vi "Read Gates From Registry (Internal).vi"(8 "error in (no error)":errorcluster, 9 "dt (us)":dbl, 10 "CMD LUT":variant, 11 "Test No.":u32) -> (0 "error out":errorcluster, 2 "Gates":T1={"Display Gate"={"Start"=0.0, "Length"=100.0}, "ETM Mode"=enum."Echo Trigger OFF", "Echo Gate"={"Start (us)"=0.0, "Length (us)"=100.0, "Threshold"=10, "Colour"=0}, "Insp Gates"=[]} {"Insp Gates"."Max # Peaks" max=64000 step=100; "Insp Gates"."Threshold" min=10 max=4095 step=10; "Insp Gates"."Length (us)" min=0.0 max=96000.0 step=100.0; "Insp Gates"."Start (us)" min=0.0 max=64000.0 step=100.0; "Echo Gate"."Threshold" min=10 max=4095 step=10; "Echo Gate"."Length (us)" min=0.0 max=96000.0 step=100.0; "Echo Gate"."Start (us)" min=0.0 max=64000.0 step=100.0; "Display Gate"."Length" min=0.0 max=64000.0 step=1000.0; "Display Gate"."Start" min=0.0 max=64000.0 step=1000.0})   [LabVIEW 2026, in "MicroPulse_Driver.lvlib"]
uses:
  MicroPulse_Driver.lvlib
  Public/Data/Datatypes/subdatatypes/MP - Registry Gates.ctl
  Public/Data/Datatypes/MP - display gate.ctl
  Public/Data/Datatypes/MP - echo gate mode.ctl
  Public/Data/Datatypes/MP - echo gate parameters.ctl
  Public/Data/Datatypes/MP - multigate inspection gate parameters.ctl
  Public/Data/Datatypes/MP - hysteresis level.ctl
  Public/Data/Datatypes/MP - multigate mode.ctl
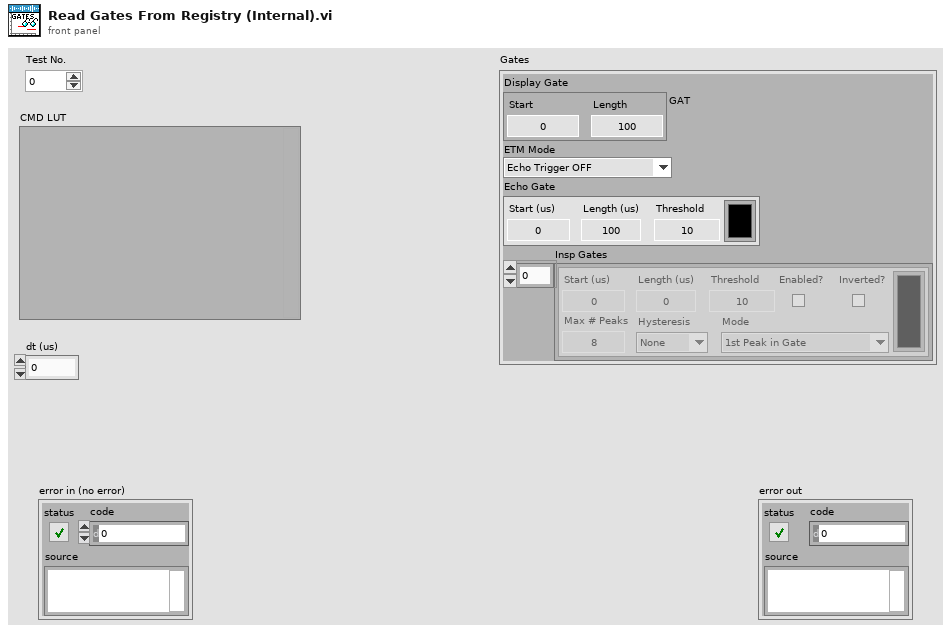
[diagram p1: front panel]
types:
  T1 = typedef "MicroPulse_Driver.lvlib/MP - Registry Gates.ctl" = cluster{"Display Gate":T2, "ETM Mode":T3, "Echo Gate":T4, "Insp Gates":T5[]}
  T2 = typedef "MicroPulse_Driver.lvlib/MP - display gate.ctl" = cluster{"Start":dbl, "Length":dbl}
  T3 = typedef "MicroPulse_Driver.lvlib/MP - echo gate mode.ctl" = enum16{"Echo Trigger OFF", "Echo Gate Display Mode", "Echo Trigger ON", "Multi Gate or FMC Mode", "Reserved", "PA - Echo Trigger ON"}
  T4 = typedef "MicroPulse_Driver.lvlib/MP - echo gate parameters.ctl" = cluster{"Start (us)":dbl, "Length (us)":dbl, "Threshold":u16, "Colour":u32}
  T5 = typedef "MicroPulse_Driver.lvlib/MP - multigate inspection gate parameters.ctl" = cluster{"Start (us)":dbl, "Length (us)":dbl, "Threshold":u16, "Enabled?":bool, "Max # Peaks":u16, "Hysteresis":T6, "Mode":T7, "Inverted?":bool, "Colour ":u32}
  T6 = typedef "MicroPulse_Driver.lvlib/MP - hysteresis level.ctl" = enum16{"None", "3dB", "6dB", "9dB", "12dB"}
  T7 = typedef "MicroPulse_Driver.lvlib/MP - multigate mode.ctl" = enum16{"1st Peak in Gate", "Largest Peak In Gate", "All Peaks In Gate", "1st Threshold Crossing"}
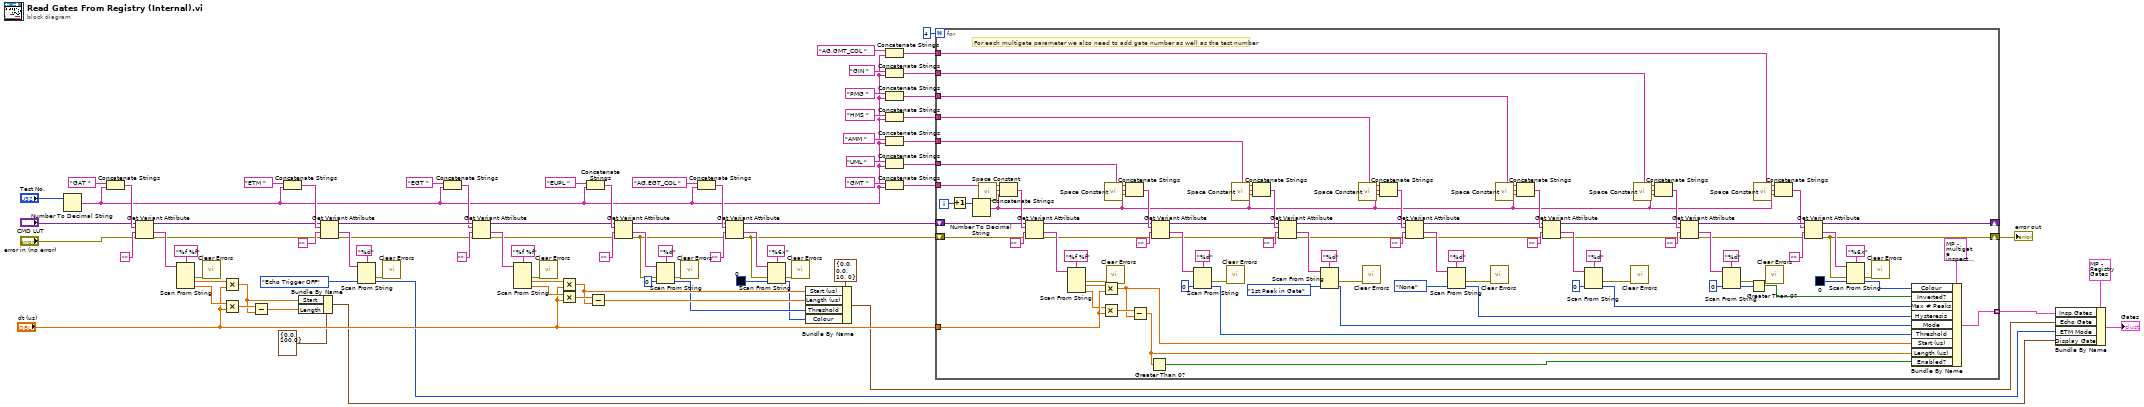
[diagram p0: block diagram]
diagram:
  n1 = Number To Decimal String(number="Test No.") -> (decimal integer string=w6:string)  [unwired: 1 in]
  n2 = Concatenate Strings("GAT " ("name"), w6) -> (w32:string)
  n3 = Get Variant Attribute(Variant="CMD LUT", name=w32, default value (empty Variant)="", error in="error in (no error)") -> (duplicate Variant=w16:variant, value=w34:string, error out=w18:errorcluster)  [unwired: 1 out]
  n4 = Scan From String(format string="%f %f", input string=w34) -> (error out=w38:errorcluster, output 1=w35:dbl, output 2=w36:dbl)  [unwired: 4 in, 2 out]
  n5 = call <vilib>:"Clear Errors.vi"("error in (no error)"=w38) -> ()  [unwired: 5 in, 2 out]
  n6 = Multiply(x=w35, y="dt (us)") -> (x*y=w27:dbl)
  n7 = Multiply(x=w36, y="dt (us)") -> (x*y=w37:dbl)
  n8 = Subtract(x=w37, y=w27) -> (x-y=w26:dbl)
  n9 = Concatenate Strings("ETM " ("name"), w6) -> (w76:string)
  n10 = Bundle By Name(cluster=T2 {"Start"=0.0, "Length"=100.0} ("Display Gate"), "Start"=w27, "Length"=w26) -> (w20:T2)
  n11 = Get Variant Attribute(Variant=w16, name=w76, default value (empty Variant)="", error in=w18) -> (duplicate Variant=w79:variant, value=w82:string, error out=w41:errorcluster)  [unwired: 1 out]
  n12 = Scan From String(format string="%d", input string=w82, default 1=MP_-_echo_gate_mode."Echo Trigger OFF" ("Echo Gate Mode")) -> (error out=w40:errorcluster, output 1=w21:T3)  [unwired: 2 in, 2 out]
  n13 = call <vilib>:"Clear Errors.vi"("error in (no error)"=w40) -> ()  [unwired: 5 in, 2 out]
  n14 = Concatenate Strings("EGT " ("name"), w6) -> (w74:string)
  n15 = Get Variant Attribute(Variant=w79, name=w74, default value (empty Variant)="", error in=w41) -> (duplicate Variant=w58:variant, value=w72:string, error out=w42:errorcluster)  [unwired: 1 out]
  n16 = Scan From String(format string="%f %f", input string=w72) -> (error out=w39:errorcluster, output 1=w65:dbl, output 2=w64:dbl)  [unwired: 4 in, 2 out]
  n17 = call <vilib>:"Clear Errors.vi"("error in (no error)"=w39) -> ()  [unwired: 5 in, 2 out]
  n18 = Multiply(x=w65, y="dt (us)") -> (x*y=w60:dbl)
  n19 = Multiply(x=w64, y="dt (us)") -> (x*y=w63:dbl)
  n20 = Concatenate Strings("EUPL " ("name"), w6) -> (w69:string)
  n21 = Subtract(x=w63, y=w60) -> (x-y=w61:dbl)
  n22 = Get Variant Attribute(Variant=w58, name=w69, default value (empty Variant)="", error in=w42) -> (duplicate Variant=w4:variant, value=w71:string, error out=w2:errorcluster)  [unwired: 1 out]
  n23 = Scan From String(format string="%d", input string=w71, error in=w2, default 1=u16 0 ("default value 1")) -> (error out=w54:errorcluster, output 1=w59:u16)  [unwired: 1 in, 2 out]
  n24 = call <vilib>:"Clear Errors.vi"("error in (no error)"=w54) -> ()  [unwired: 5 in, 2 out]
  n25 = Concatenate Strings("AG.EGT_COL " ("name"), w6) -> (w12:string)
  n26 = Get Variant Attribute(Variant=w4, name=w12, default value (empty Variant)="", error in=w2) -> (duplicate Variant=w3:variant, value=w10:string, error out=w1:errorcluster)  [unwired: 1 out]
  n27 = Scan From String(format string="%6x", input string=w10, error in=w1, default 1=u32 0 ("Color Box")) -> (error out=w15:errorcluster, output 1=w9:u32)  [unwired: 1 in, 2 out]
  n28 = call <vilib>:"Clear Errors.vi"("error in (no error)"=w15) -> ()  [unwired: 5 in, 2 out]
  n29 = Bundle By Name(cluster=T4 {"Start (us)"=0.0, "Length (us)"=0.0, "Threshold"=10, "Colour"=0} ("Echo Gate Parameters"), "Start (us)"=w60, "Length (us)"=w61, "Threshold"=w59, "Colour"=w9) -> (w22:T4)
  n30 = Concatenate Strings("AG.GMT_COL " ("name"), w6) -> (w5:string)
  n31 = Concatenate Strings("GIN " ("name"), w6) -> (w44:string)
  n32 = Concatenate Strings("PMG " ("name"), w6) -> (w45:string)
  n33 = Concatenate Strings("HMS " ("name"), w6) -> (w46:string)
  n34 = Concatenate Strings("AMM " ("name"), w6) -> (w50:string)
  n35 = Concatenate Strings("UML " ("name"), w6) -> (w52:string)
  n36 = Concatenate Strings("GMT " ("name"), w6) -> (w56:string)
  n37 = for {
    N: 4 -> [_]
    tunnel: w56 -> [w173]
    shift-right: [w92] -> _
    shift-left: w3 -> [w166]
    shift-right: [w90] -> w43
    shift-left: w1 -> [w165]
    tunnel: "dt (us)" -> [w162]
    tunnel: w52 -> [w155]
    tunnel: w50 -> [w147]
    tunnel: w46 -> [w123]
    tunnel: w45 -> [w122]
    tunnel: w44 -> [w121]
    tunnel: [w110] -> w23 mode=indexing
    tunnel: w5 -> [w85]
    i -> [w169]
    # "For each multigate parameter we also need to add gate number as well as the test number"
    n38 = Increment(x=w169) -> (x+1=w168:i32)
    n39 = Number To Decimal String(number=w168) -> (decimal integer string=w86:string)  [unwired: 1 in]
    n40 = call <vilib>:"Space Constant.vi"() -> ("String"=w167:string)
    n41 = Concatenate Strings(w173, w167, w86) -> (w170:string)
    n42 = Get Variant Attribute(Variant=w166, name=w170, default value (empty Variant)="", error in=w165) -> (duplicate Variant=w154:variant, value=w171:string, error out=w109:errorcluster)  [unwired: 1 out]
    n43 = Scan From String(format string="%f %f", input string=w171) -> (error out=w108:errorcluster, output 1=w163:dbl, output 2=w161:dbl)  [unwired: 4 in, 2 out]
    n44 = Multiply(x=w163, y=w162) -> (x*y=w111:dbl)
    n45 = Multiply(x=w161, y=w162) -> (x*y=w164:dbl)
    n46 = call <vilib>:"Space Constant.vi"() -> ("String"=w160:string)
    n47 = call <vilib>:"Clear Errors.vi"("error in (no error)"=w108) -> ()  [unwired: 5 in, 2 out]
    n48 = Concatenate Strings(w155, w160, w86) -> (w156:string)
    n49 = Subtract(x=w164, y=w111) -> (x-y=w112:dbl)
    n50 = Greater Than 0?(x=w112) -> (x > 0?=w113:bool)
    n51 = Get Variant Attribute(Variant=w154, name=w156, default value (empty Variant)="", error in=w109) -> (duplicate Variant=w145:variant, value=w159:string, error out=w100:errorcluster)  [unwired: 1 out]
    n52 = Scan From String(format string="%d", input string=w159, default 1=u16 0 ("default value 1")) -> (error out=w99:errorcluster, output 1=w114:u16)  [unwired: 2 in, 2 out]
    n53 = call <vilib>:"Clear Errors.vi"("error in (no error)"=w99) -> ()  [unwired: 5 in, 2 out]
    n54 = call <vilib>:"Space Constant.vi"() -> ("String"=w148:string)
    n55 = Concatenate Strings(w147, w148, w86) -> (w152:string)
    n56 = Get Variant Attribute(Variant=w145, name=w152, default value (empty Variant)="", error in=w100) -> (duplicate Variant=w127:variant, value=w149:string, error out=w102:errorcluster)  [unwired: 1 out]
    n57 = Scan From String(format string="%d", input string=w149, default 1=MP_-_multigate_mode."1st Peak in Gate" ("Value")) -> (error out=w101:errorcluster, output 1=w115:T7)  [unwired: 2 in, 2 out]
    n58 = call <vilib>:"Space Constant.vi"() -> ("String"=w140:string)
    n59 = call <vilib>:"Clear Errors.vi"("error in (no error)"=w101) -> ()  [unwired: 5 in, 2 out]
    n60 = Concatenate Strings(w123, w140, w86) -> (w144:string)
    n61 = Get Variant Attribute(Variant=w127, name=w144, default value (empty Variant)="", error in=w102) -> (duplicate Variant=w126:variant, value=w141:string, error out=w104:errorcluster)  [unwired: 1 out]
    n62 = Scan From String(format string="%d", input string=w141, default 1=MP_-_hysteresis_level."None" ("Value")) -> (error out=w103:errorcluster, output 1=w116:T6)  [unwired: 2 in, 2 out]
    n63 = call <vilib>:"Clear Errors.vi"("error in (no error)"=w103) -> ()  [unwired: 5 in, 2 out]
    n64 = call <vilib>:"Space Constant.vi"() -> ("String"=w139:string)
    n65 = Concatenate Strings(w122, w139, w86) -> (w135:string)
    n66 = Get Variant Attribute(Variant=w126, name=w135, default value (empty Variant)="", error in=w104) -> (duplicate Variant=w125:variant, value=w138:string, error out=w106:errorcluster)  [unwired: 1 out]
    n67 = Scan From String(format string="%d", input string=w138, default 1=u16 0 ("default value 1")) -> (error out=w105:errorcluster, output 1=w117:u16)  [unwired: 2 in, 2 out]
    n68 = call <vilib>:"Clear Errors.vi"("error in (no error)"=w105) -> ()  [unwired: 5 in, 2 out]
    n69 = call <vilib>:"Space Constant.vi"() -> ("String"=w128:string)
    n70 = Concatenate Strings(w121, w128, w86) -> (w132:string)
    n71 = Get Variant Attribute(Variant=w125, name=w132, default value (empty Variant)="", error in=w106) -> (duplicate Variant=w93:variant, value=w129:string, error out=w91:errorcluster)  [unwired: 1 out]
    n72 = Scan From String(format string="%d", input string=w129, default 1=u16 0 ("default value 1")) -> (error out=w107:errorcluster, output 1=w119:u16)  [unwired: 2 in, 2 out]
    n73 = Greater Than 0?(x=w119) -> (x > 0?=w118:bool)
    n74 = call <vilib>:"Space Constant.vi"() -> ("String"=w88:string)
    n75 = call <vilib>:"Clear Errors.vi"("error in (no error)"=w107) -> ()  [unwired: 5 in, 2 out]
    n76 = Concatenate Strings(w85, w88, w86) -> (w87:string)
    n77 = Get Variant Attribute(Variant=w93, name=w87, default value (empty Variant)="", error in=w91) -> (duplicate Variant=w92:variant, value=w95:string, error out=w90:errorcluster)  [unwired: 1 out]
    n78 = Scan From String(format string="%6x", input string=w95, error in=w90, default 1=u32 0 ("Color Box")) -> (error out=w98:errorcluster, output 1=w89:u32)  [unwired: 1 in, 2 out]
    n79 = call <vilib>:"Clear Errors.vi"("error in (no error)"=w98) -> ()  [unwired: 5 in, 2 out]
    n80 = Bundle By Name(cluster=T5 {"Start (us)"=0.0, "Length (us)"=0.0, "Threshold"=0, "Enabled?"=FALSE, "Max # Peaks"=0, "Hysteresis"=enum."None", "Mode"=enum."1st Peak in Gate", "Inverted?"=FALSE, "Colour "=0} ("Gate 1"), "Colour"=w89, "Inverted?"=w118, "Max # Peaks"=w117, "Hysteresis"=w116, "Mode"=w115, "Threshold"=w114, "Start (us)"=w111, "Length (us)"=w112, "Enabled?"=w113) -> (w110:T5)
  }
  "error out" <- w43
  n81 = Bundle By Name(cluster=T1 {"Display Gate"={"Start"=0.0, "Length"=100.0}, "ETM Mode"=enum."Echo Trigger OFF", "Echo Gate"={"Start (us)"=0.0, "Length (us)"=100.0, "Threshold"=10, "Colour"=0}, "Insp Gates"=[]} ("Gates"), "Insp Gates"=w23, "Echo Gate"=w22, "ETM Mode"=w21, "Display Gate"=w20) -> (→"Gates":T1)
